vi "_ViewInFolder.vi"(6 "Variant in":variant, 8 "error in (no error)":errorcluster, 9 "Shift Pressed?":bool, 10 "QD Combo Box Ref":refnum<vi>, 11 "QD Launch VI Ref":refnum<vi>) -> (0 "error out":errorcluster, 4 "Variant out":variant)   [LabVIEW 2014, in "NEVSTOP QD Shortcuts.lvlib"]
uses:
  NEVSTOP QD Shortcuts.lvlib
panel:
  # "Do not change the connector pane of this VI.\n\nSee the block diagram for directions on how to use this template."
  # "Specify the name of the Undo transaction"
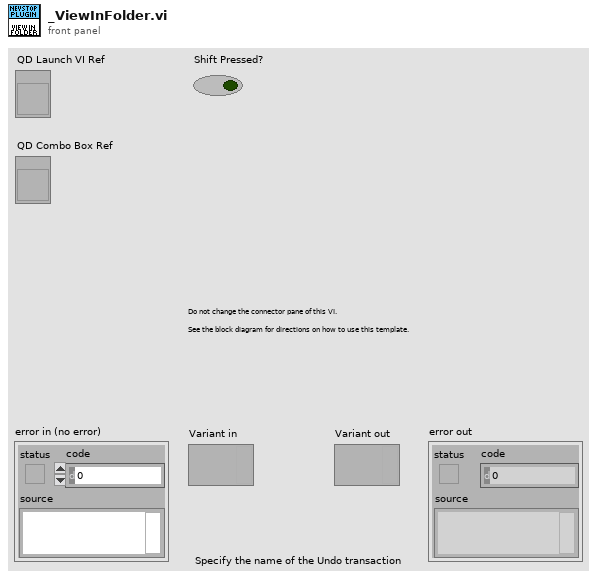
[diagram p1: front panel]
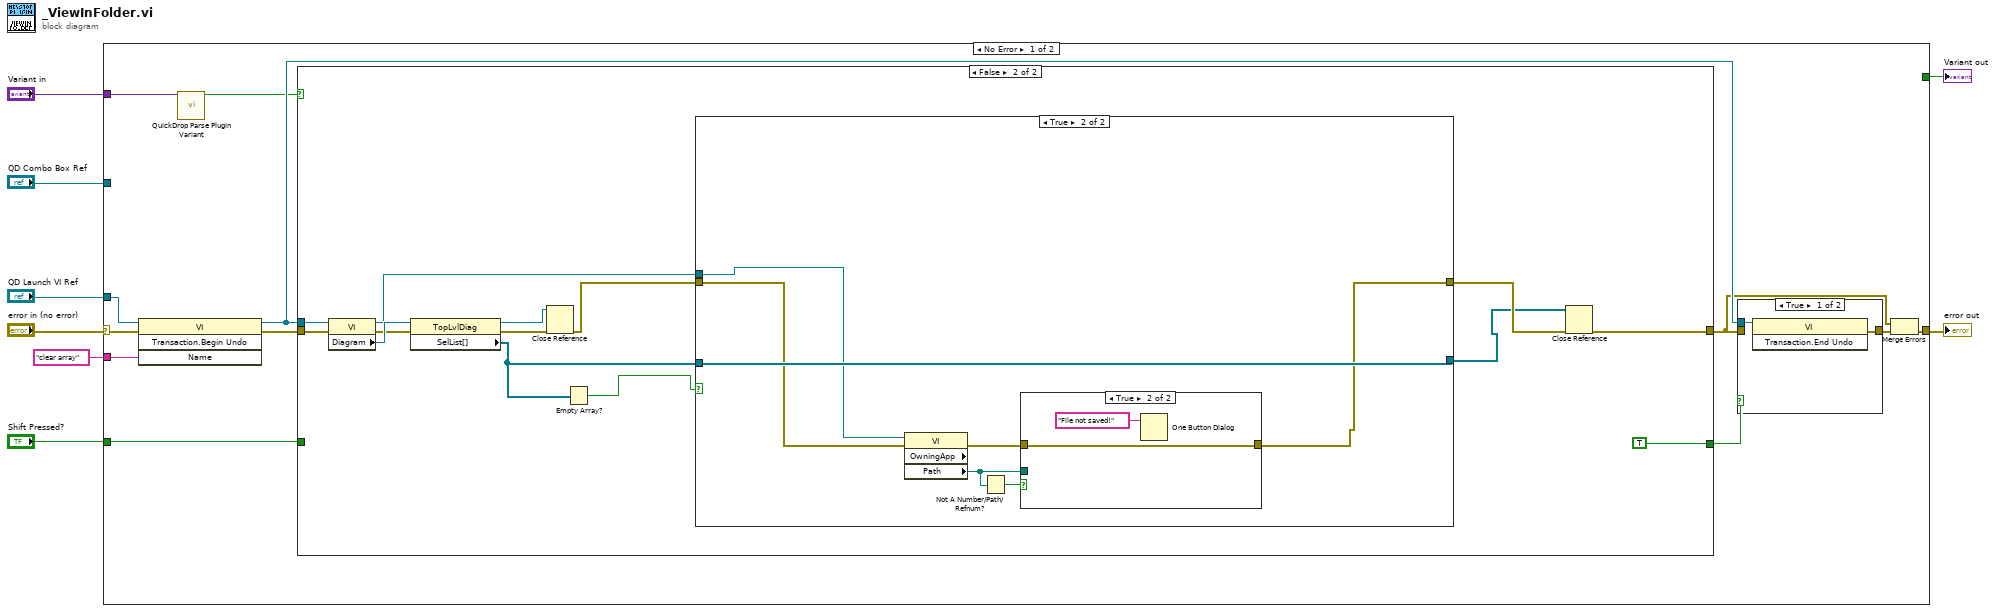
[diagram p0: block diagram]
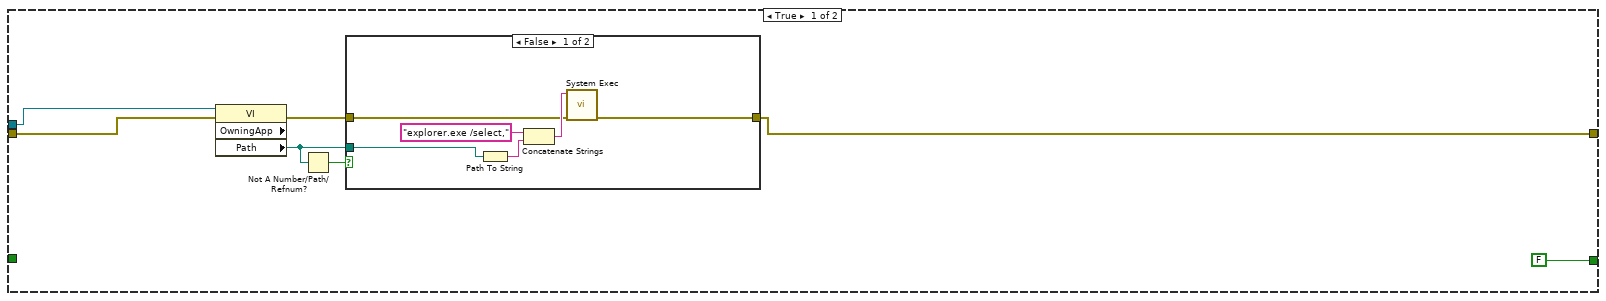
[diagram p2: hidden frame]
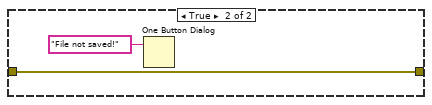
[diagram p3: hidden frame]
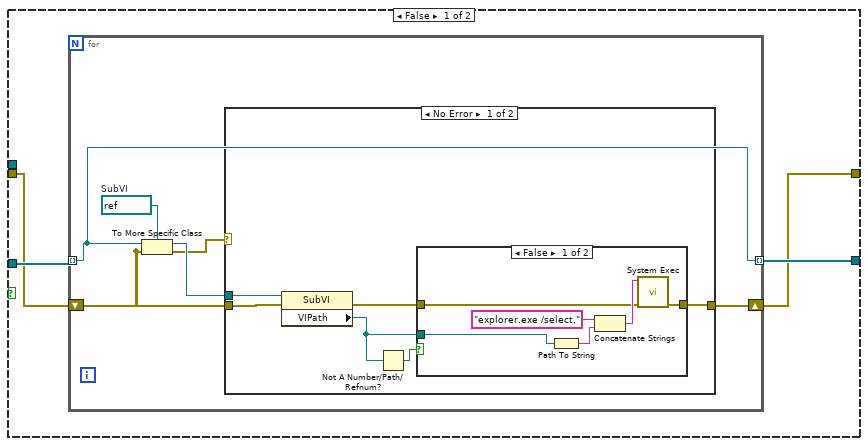
[diagram p4: hidden frame]
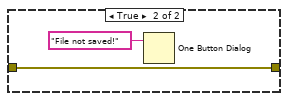
[diagram p5: hidden frame]
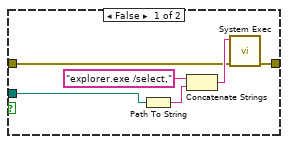
[diagram p7: hidden frame]
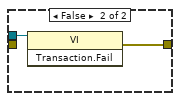
[diagram p8: hidden frame]
diagram:
  n1 = case shown="No Error" "error in (no error)" {
    selector: "error in (no error)" -> [w20 w95]
    tunnel: [w10 w95] -> w7
    tunnel: "QD Launch VI Ref" -> [w19 _]
    tunnel: "Shift Pressed?" -> [w14 _]
    tunnel: "QD Combo Box Ref" -> [_ _]
    tunnel: "Variant in" -> [w21 _]
    tunnel: "clear array" ("Undo Name") -> [w18 _]
    tunnel: [TRUE _] -> w1
    frame No Error {
      n2 = invoke class="VI" method="Transaction.Begin Undo"(reference=w19, error in=w20, "Name"=w18) -> (reference out=w13:refnum<vi>, error out=w16:errorcluster)  [unwired: 1 in, 2 out]
      n3 = call <vilib>:"QuickDrop Parse Plugin Variant.vi"("QDKS Variant in"=w21) -> ("QD Launch VI Panel?"=w12:bool)  [unwired: 12 in, 2 out]
      n4 = case shown="False" w12 {
        tunnel: w16 -> [w23 w50]
        tunnel: [w22 w48] -> w9
        tunnel: w14 -> [_ _]
        tunnel: w13 -> [w24 w47]
        tunnel: [FALSE TRUE] -> w11
        frame True {
          n5 = property class="VI" props=["OwningApp", "Path"](reference=w24, error in=w23) -> (error out=w26:errorcluster, "Path"=w25:path)  [unwired: 2 out]
          n6 = Not A Number/Path/Refnum?(number/path/refnum=w25) -> (NaN/Path/Refnum?=w27:bool)
          n7 = case shown="False" w27 {
            tunnel: [w31 w36] -> w22
            tunnel: w26 -> [w30 w36]
            tunnel: w25 -> [w29 _]
            frame False {
              n8 = Path To String(path=w29) -> (string=w33:string)
              n9 = Concatenate Strings("explorer.exe /select,", w33) -> (w32:string)
              n10 = call <vilib>:"System Exec.vi"("error in (no error)"=w30, "command line"=w32) -> ("error out"=w31:errorcluster)  [unwired: 6 in, 3 out]
            }
            frame True {
              n11 = One Button Dialog(message="File not saved!") -> ()  [unwired: 1 in, 1 out]
            }
          }
        }
        frame False {
          n12 = property class="VI"(reference=w47, error in=w50) -> (reference out=w40:refnum<vi>, error out=w45:errorcluster, "Diagram"=w46:refnum<vi>)
          n13 = property class="TopLvlDiag"(reference=w46, error in=w45) -> (reference out=w43:refnum<vi>, error out=w49:errorcluster, "SelList[]"=w38:refnum<vi>[])
          n14 = Close Reference(reference=w43, error in (no error)=w49) -> (error out=w41:errorcluster)
          n15 = Empty Array?(array=w38) -> (empty?=w42:bool)
          n16 = case shown="True" w42 {
            tunnel: w41 -> [w52 w77]
            tunnel: w40 -> [_ w78]
            tunnel: [w51 w76] -> w39
            tunnel: w38 -> [w54 w82]
            tunnel: [w53 w82] -> w37
            frame False {
              n17 = for {
                tunnel: w54 -> [w58] mode=indexing
                tunnel: [w58] -> w53 mode=indexing
                shift-right: [w55] -> w51
                shift-left: w52 -> [w56]
                w60 = refnum<vi> refnum  # SubVI
                n18 = To More Specific Class(target class=w60, reference=w58, error in=w56) -> (specific class reference=w59:refnum<vi>, error out=w57:errorcluster)
                n19 = case shown="No Error" w57 {
                  tunnel: w59 -> [w63 _]
                  tunnel: w56 -> [w62 w75]
                  tunnel: [w61 w75] -> w55
                  frame No Error {
                    n20 = property on="Property Node" class="SubVI"(reference=w63, error in=w62) -> (error out=w65:errorcluster, "VIPath"=w66:path)  [unwired: 1 out]
                    n21 = Not A Number/Path/Refnum?(number/path/refnum=w66) -> (NaN/Path/Refnum?=w64:bool)
                    n22 = case shown="False" w64 {
                      tunnel: [w69 w74] -> w61
                      tunnel: w65 -> [w68 w74]
                      tunnel: w66 -> [w67 _]
                      frame False {
                        n23 = Path To String(path=w67) -> (string=w71:string)
                        n24 = Concatenate Strings("explorer.exe /select,", w71) -> (w70:string)
                        n25 = call <vilib>:"System Exec.vi"("error in (no error)"=w68, "command line"=w70) -> ("error out"=w69:errorcluster)  [unwired: 6 in, 3 out]
                      }
                      frame True {
                        n26 = One Button Dialog(message="File not saved!") -> ()  [unwired: 1 in, 1 out]
                      }
                    }
                  }
                  frame Error {
                  }
                }
              }
            }
            frame True {
              n27 = property on="Property Node" class="VI" props=["OwningApp", "Path"](reference=w78, error in=w77) -> (error out=w80:errorcluster, "Path"=w81:path)  [unwired: 2 out]
              n28 = Not A Number/Path/Refnum?(number/path/refnum=w81) -> (NaN/Path/Refnum?=w79:bool)
              n29 = case shown="True" w79 {
                tunnel: [w85 w90] -> w76
                tunnel: w80 -> [w84 w90]
                tunnel: w81 -> [w83 _]
                frame False {
                  n30 = Path To String(path=w83) -> (string=w87:string)
                  n31 = Concatenate Strings("explorer.exe /select,", w87) -> (w86:string)
                  n32 = call <vilib>:"System Exec.vi"("error in (no error)"=w84, "command line"=w86) -> ("error out"=w85:errorcluster)  [unwired: 6 in, 3 out]
                }
                frame True {
                  n33 = One Button Dialog(message="File not saved!") -> ()  [unwired: 1 in, 1 out]
                }
              }
            }
          }
          n34 = Close Reference(reference=w37, error in (no error)=w39) -> (error out=w48:errorcluster)
        }
      }
      n35 = case shown="True" w11 {
        tunnel: w13 -> [w91 w93]
        tunnel: [w92 w94] -> w15
        tunnel: w9 -> [_ _]
        frame True {
          n36 = invoke class="VI" method="Transaction.End Undo"(reference=w91) -> (error out=w92:errorcluster)  [unwired: 2 in, 2 out]
        }
        frame False {
          n37 = invoke class="VI" method="Transaction.Fail"(reference=w93) -> (error out=w94:errorcluster)  [unwired: 2 in, 2 out]
        }
      }
      n38 = Merge Errors(w9, w15) -> (w10:errorcluster)
    }
    frame Error {
    }
  }
  "error out" <- w7
  "Variant out" <- w1
